vi "Send Data.vi"(7 "Finished Late":bool, 8 "error in (no error)":errorcluster, 11 "ValveControlModule in":refnum<class "DigitalControlModule.lvclass">) -> (0 "error out":errorcluster, 3 "ValveControlModule out":refnum<class "DigitalControlModule.lvclass">)   [LabVIEW 2020, in "VolatusControl.lvlib" / "DigitalControlModule.lvclass"]
uses:
  DigitalControlModule.lvclass
  DigitalControlModule.lvclass/DigitalControlModule.ctl
  VolatusData/VolatusData.lvlib
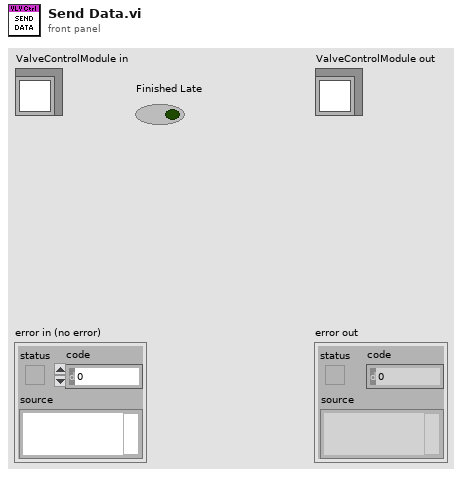
[diagram p1: front panel]
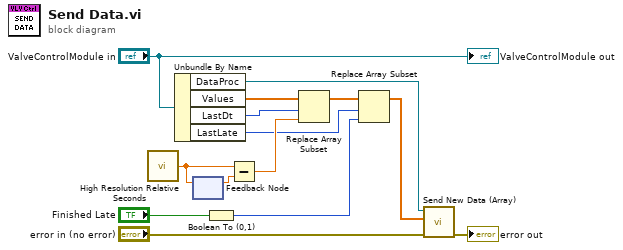
[diagram p0: block diagram]
diagram:
  n1 = call <vilib>:"High Resolution Relative Seconds.vi"() -> ("relative seconds"=w8:dbl)
  n2 = Unbundle By Name("ValveControlModule in") -> ("DataProc"=w13:refnum<class "MessageQ.lvclass">, "Values"=w12:dbl[], "LastDt"=w5:i32, "LastLate"=w2:i32)
  n3 = feedback #1() -> (w9:dbl)  [unwired: 1 in]
  n4 = feedback-in #1(w8) -> ()
  n5 = Boolean To (0,1)(Boolean="Finished Late") -> (0, 1=w1:i16)
  n6 = Subtract(x=w8, y=w9) -> (x-y=w4:dbl)
  n7 = Replace Array Subset(array=w12, new element=w4, index=w5) -> (w6:dbl[])
  n8 = Replace Array Subset(array=w6, new element=w1, index=w2) -> (w3:dbl[])
  n9 = call "Send New Data (Array).vi"("error in (no error)"="error in (no error)", "Data"=w3, "MessageQ"=w13) -> ("error out"=→"error out":errorcluster)  [unwired: 8 in]
  "ValveControlModule out" <- "ValveControlModule in"
